vi "Move Needle Impl.vi"(8 "error in (no error)":errorcluster, 10 "Needle Position":T1, 11 "Simulated Autosampler in":refnum<class "Simulated Autosampler.lvclass">) -> (0 "error out":errorcluster, 3 "Simulated Autosampler out":refnum<class "Simulated Autosampler.lvclass">)   [LabVIEW 2023, in "Simulated Autosampler.lvlib" / "Simulated Autosampler.lvclass"]
uses:
  Simulated Autosampler.lvclass
  Autosampler/Autosampler Needle Position.ctl
  Simulated Autosampler.lvclass/Simulated Autosampler.ctl
  Autosampler/Autosampler.lvlib
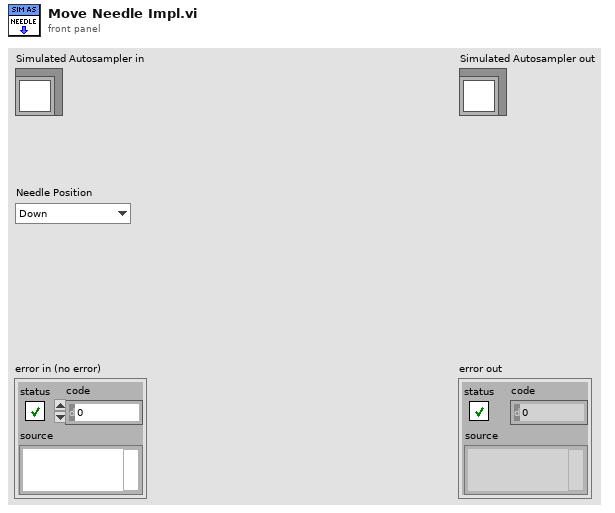
[diagram p1: front panel]
types:
  T1 = typedef "Autosampler.lvlib/Autosampler Needle Position.ctl" = enum16{"Down", "Up"}
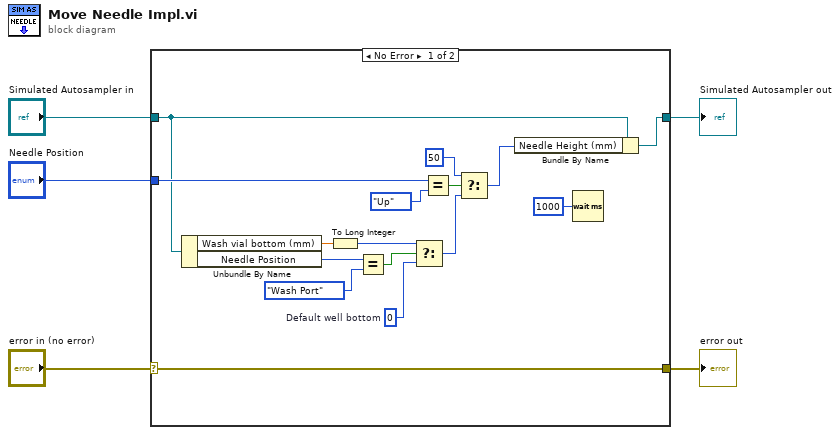
[diagram p0: block diagram]
diagram:
  n1 = case shown="No Error" "error in (no error)" {
    selector: "error in (no error)" -> [w11 w23]
    tunnel: [w11 w23] -> w4
    tunnel: "Simulated Autosampler in" -> [w14 w22]
    tunnel: [w20 w22] -> w2
    tunnel: "Needle Position" -> [w18 _]
    frame No Error {
      w12 = 0  # Default well bottom
      n2 = Unbundle By Name(w14) -> ("Wash vial bottom (mm)"=w13:dbl, "Needle Position"=w9:enum16{"Home", "Well", "Wash Port"})
      n3 = To Long Integer(number=w13) -> (32bit integer=w10:i32)
      n4 = Equal?(x=w9, y=enum16{"Home", "Well", "Wash Port"}."Wash Port") -> (x = y?=w8:bool)
      n5 = Select(t=w10, s=w8, f=w12) -> (s? t:f=w6:i32)
      n6 = Equal?(x=w18, y=Autosampler_Needle_Position."Up") -> (x = y?=w19:bool)
      n7 = Select(t=50 ("f"), s=w19, f=w6) -> (s? t:f=w15:i32)
      n8 = Bundle By Name(cluster=w14, "Needle Height (mm)"=w15) -> (w20:refnum<class "Simulated Autosampler.lvclass">)
      n9 = Wait (ms)(milliseconds to wait=u32 1000) -> ()  [unwired: 1 out]
    }
    frame Error {
    }
  }
  "error out" <- w4
  "Simulated Autosampler out" <- w2
